vi "single action.vi"() -> ()   [LabVIEW 2013]
uses:
  result/result.lvclass
  dispatcher/pool sizes.ctl
  result/result.lvclass/result.ctl
  result/get data.vi
  result/get error.vi
  result/get owning task.vi
  result/get subresults.vi
  dispatcher/thread pool.lvclass
  standard reporters/event reporter/event reporter.lvclass
  standard action/wait action/wait action.lvclass
panel:
  out "x-y 2":dbl
  out "x-y":dbl
  out "subresults":refnum<class "result.lvclass">[](array[class])
  out "owning task":string
  out "error":errorcluster
  out "data":variant
  out "Time":u32
  out "result":refnum<class "result.lvclass">
  out "error out":errorcluster
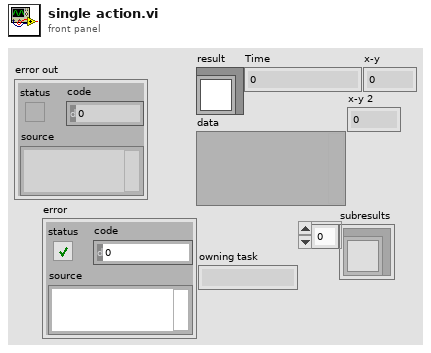
[diagram p1: front panel]
types:
  T1 = typedef "thread pool.lvclass/pool sizes.ctl" = cluster{"UI thread":u8, "standard":u8, "instrument I/O":u8, "data acquisition":u8, "other 1":u8, "other 2":u8}
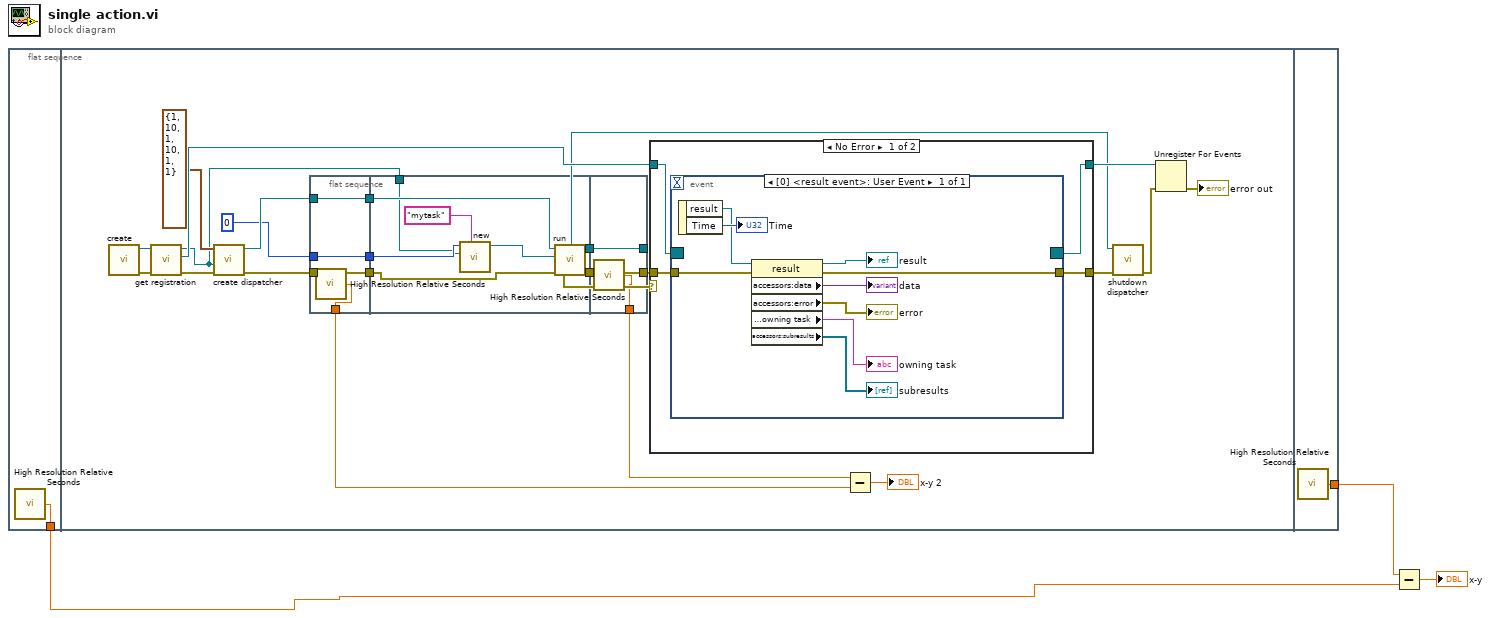
[diagram p0: block diagram]
diagram:
  n1 = flat-sequence {
    tunnel: [w4] -> w2
    tunnel: [w58] -> w3
    frame #0 {
      n2 = call <vilib>:"High Resolution Relative Seconds.vi"() -> ("relative seconds"=w4:dbl)
    }
    frame #1 {
      n3 = call "create.vi"() -> ("error out"=w23:errorcluster, "event reporter out"=w24:refnum<class "event reporter.lvclass">)  [unwired: 10 in]
      n4 = call "get registration.vi"("error in"=w23, "event reporter in"=w24) -> ("error out"=w22:errorcluster, "result registration"=w21:refnum<event-registration>, "event reporter out"=w5:refnum<class "event reporter.lvclass">)  [unwired: 7 in]
      n5 = call "create dispatcher.vi"("error in"=w22, "default reporter"=w5, "initial pool sizes"=T1 {"UI thread"=1, "standard"=10, "instrument I/O"=1, "data acquisition"=10, "other 1"=1, "other 2"=1}) -> ("error out"=w26:errorcluster, "dispatcher"=w27:refnum<data-value>)  [unwired: 7 in]
      n6 = flat-sequence {
        tunnel: 0 -> [w29]
        tunnel: w26 -> [w30]
        tunnel: w27 -> [w31]
        tunnel: [w31] -> w11
        tunnel: [w30] -> w10
        tunnel: [w29] -> w9
        tunnel: [w28] -> w7
        tunnel: [w38] -> w13
        tunnel: [w37] -> w12
        tunnel: w11 -> [w39]
        tunnel: w10 -> [w35]
        tunnel: w9 -> [w34]
        tunnel: w5 -> [w32]
        tunnel: [w41] -> w15
        tunnel: [w42] -> w19
        tunnel: w13 -> [w42]
        tunnel: w12 -> [w41]
        tunnel: [w40] -> w8
        frame #0 {
          n7 = call <vilib>:"High Resolution Relative Seconds.vi"() -> ("relative seconds"=w28:dbl)
        }
        frame #1 {
          n8 = call "new.vi"("ID"="mytask", "results reporter"=w32, "timer"=w34) -> ("wait action out"=w36:refnum<class "wait action.lvclass">)  [unwired: 8 in]
          n9 = call "run.vi"("error in"=w35, "task"=w36, "dispatcher"=w39) -> ("error out"=w37:errorcluster, "dispatcher out"=w38:refnum<data-value>)  [unwired: 7 in]
        }
        frame #2 {
          n10 = call <vilib>:"High Resolution Relative Seconds.vi"() -> ("relative seconds"=w40:dbl)
        }
      }
      n11 = case shown="No Error" w15 {
        tunnel: w21 -> [w46 w57]
        tunnel: [w45 w57] -> w20
        tunnel: [w44 w56] -> w16
        tunnel: w15 -> [w43 w56]
        frame No Error {
          n12 = event shown="[0] <result event>: User Event" {
            selector: w46 -> [_]
            dyn-events: [_] -> w45
            timeout: _ -> [_]
            tunnel: [w53] -> w44
            tunnel: w43 -> [w54]
            event User Event {
              n13 = event-data() -> ("result"=w52:refnum<class "result.lvclass">, "Time"=→"Time":u32)  [unwired: 1 in]
              n14 = property class="result"(reference=w52, error in=w54) -> (reference out=→"result":refnum<class "result.lvclass">, error out=w53:errorcluster, "accessors:data"=→"data":variant, "accessors:error"=→"error":errorcluster, "accessors:owning task"=→"owning task":string, "accessors:subresults"=→"subresults":refnum<class "result.lvclass">[])
            }
          }
        }
        frame Error {
        }
      }
      n15 = Subtract(x=w8, y=w7) -> (x-y=→"x-y 2":dbl)
      n16 = call "shutdown dispatcher.vi"("error in"=w16, "dispatcher"=w19) -> ("error out"=w18:errorcluster)  [unwired: 9 in]
      n17 = Unregister For Events(event registration refnum=w20, error in=w18) -> (error out=→"error out":errorcluster)
    }
    frame #2 {
      n18 = call <vilib>:"High Resolution Relative Seconds.vi"() -> ("relative seconds"=w58:dbl)
    }
  }
  n19 = Subtract(x=w3, y=w2) -> (x-y=→"x-y":dbl)
